vi "FIND_MOD_NAMES.vi"(11 "RICERCA cDAQ":string="NICOTRA") -> (0 "error out":errorcluster, 1 "Array REF":refnum<k20>[](array[refnum]), 2 "Array ALIAS":string[](array[string]), 3 "Array nomi moduli":string[](array[string]))   [LabVIEW 2019]
uses:
  <vilib>/nisyscfg/Find Hardware.vi
  <vilib>/nisyscfg/Close (System).vi
  <vilib>/nisyscfg/nisyscfg.lvlib
  <resource>/objmgr/nicontrollersysapi.rc
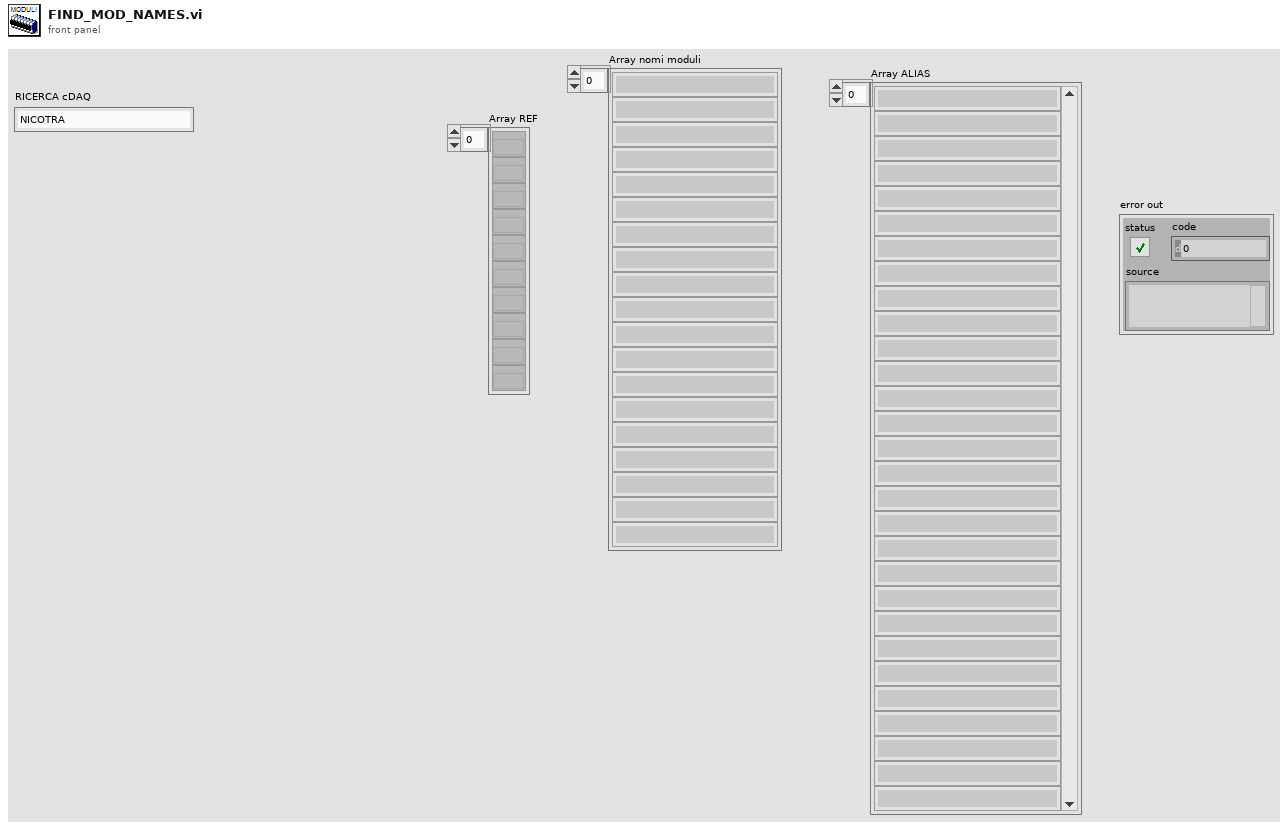
[diagram p1: front panel]
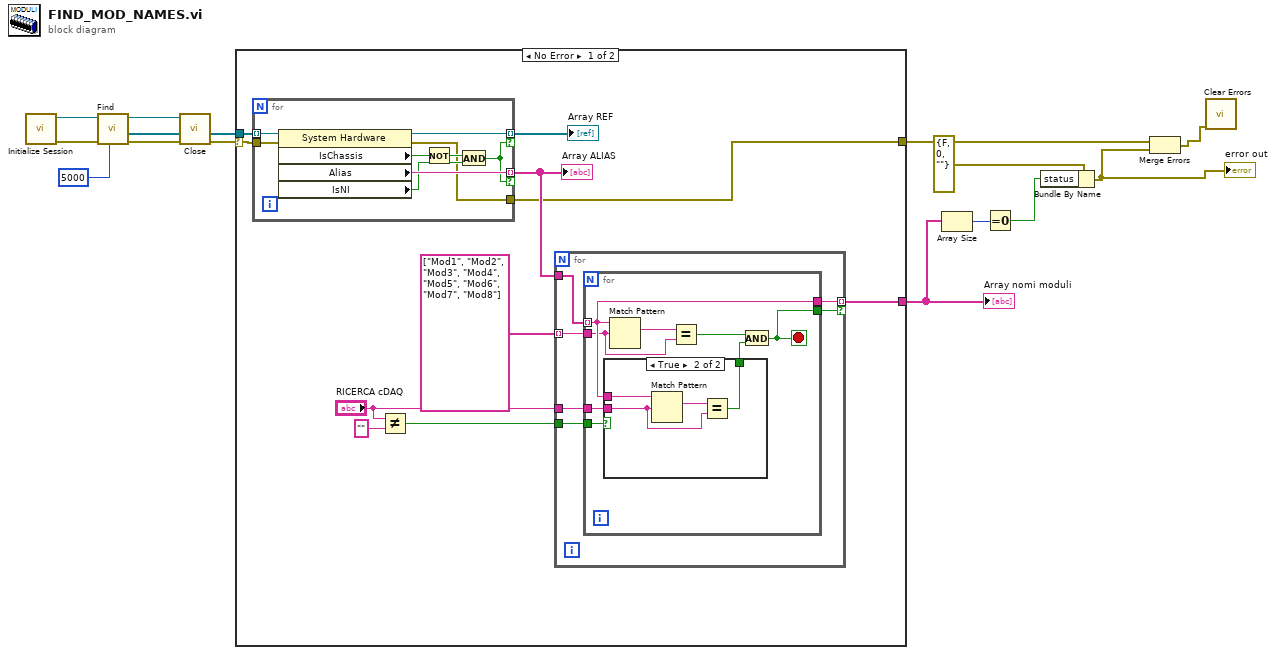
[diagram p0: block diagram]
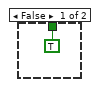
[diagram p2: hidden frame]
diagram:
  n1 = call <vilib>:"Initialize Session.vi"() -> ("error out"=w9:errorcluster, "Session out"=w11:refnum<k21>)  [unwired: 10 in]
  n2 = call-poly <vilib>:"Find.vi"("Remote Timeout (300,000 ms)"=u32 5000, "error in (no error)"=w9, "Session in"=w11) -> ("error out"=w12:errorcluster, "Resources out"=w14:refnum<k20>[], "Session out"=w13:refnum<k21>)  [unwired: 5 in, 1 out]
  n3 = call-poly <vilib>:"Close.vi"("error in (no error)"=w12, "Session in"=w13) -> ("error out"=w8:errorcluster)  [unwired: 9 in]
  n4 = case shown="No Error" w8 {
    selector: w8 -> [w16 w53]
    tunnel: w14 -> [w24 _]
    tunnel: [w20 _] -> w7
    tunnel: [w15 w53] -> w5
    frame No Error {
      n5 = for {
        tunnel: w24 -> [w52] mode=indexing
        tunnel: [w51] -> w23 mode=indexing if=w46
        tunnel: [w50] -> w21 mode=indexing if=w46
        tunnel: w16 -> [w45]
        tunnel: [w44] -> w15
        n6 = property class="System Hardware"(reference=w52, error in=w45) -> (reference out=w51:refnum<k20>, error out=w44:errorcluster, "IsChassis"=w48:bool, "Alias"=w50:string, "IsNI"=w49:bool)
        n7 = Not(x=w48) -> (.not. x?=w47:bool)
        n8 = And(x=w47, y=w49) -> (x .and. y?=w46:bool)
      }
      "Array REF" <- w23
      "Array ALIAS" <- w21
      n9 = Not Equal?(x="RICERCA cDAQ", y="") -> (x != y?=w18:bool)
      n10 = for {
        tunnel: string[] ["Mod1", "Mod2", "Mod3", "Mod4", "Mod5", "Mod6", "Mod7", "Mod8"] -> [w29] mode=indexing
        tunnel: w21 -> [w30]
        tunnel: [w28] -> w20 mode=indexing if=w27
        tunnel: w18 -> [w26]
        tunnel: "RICERCA cDAQ" -> [w25]
        n11 = for {
          tunnel: w30 -> [w37] mode=indexing
          tunnel: w29 -> [w31]
          tunnel: [w37] -> w28
          tunnel: [w34] -> w27
          tunnel: w26 -> [w38]
          tunnel: w25 -> [w36]
          stop <- w34 stop-if-true
          n12 = case shown="True" w38 {
            tunnel: w37 -> [_ w43]
            tunnel: w36 -> [_ w41]
            tunnel: [TRUE w40] -> w33
            frame False {
            }
            frame True {
              n13 = Match Pattern(string=w43, regular expression=w41) -> (match substring=w42:string)  [unwired: 1 in, 3 out]
              n14 = Equal?(x=w42, y=w41) -> (x = y?=w40:bool)
            }
          }
          n15 = Match Pattern(string=w37, regular expression=w31) -> (match substring=w32:string)  [unwired: 1 in, 3 out]
          n16 = Equal?(x=w32, y=w31) -> (x = y?=w35:bool)
          n17 = And(x=w35, y=w33) -> (x .and. y?=w34:bool)
        }
      }
    }
    frame Error {
    }
  }
  "Array nomi moduli" <- w7
  n18 = Array Size(array=w7) -> (size(s)=w6:i32)
  n19 = Equal To 0?(x=w6) -> (x = 0?=w3:bool)
  n20 = Bundle By Name(cluster=errorcluster {"status"=FALSE, "code"=0, "source"=""} ("error in"), "status"=w3) -> (w2:errorcluster)
  "error out" <- w2
  n21 = Merge Errors(w5, w2) -> (w1:errorcluster)
  n22 = call <vilib>:"Clear Errors.vi"("error in (no error)"=w1) -> ()  [unwired: 5 in, 2 out]
